vi "ScreenshotSingleVIs.vi"(6 "Title Prefix In":string, 8 "error in":errorcluster, 9 "Picture Save Location":path, 10 "New VI Path":path) -> (0 "error out":errorcluster)   [LabVIEW 2015, in "VIDiffScreenshots.lvlib"]
uses:
  VIDiffScreenshots.lvlib
  Utilities/Arguments.ctl
  VIScreenshots.ctl
  ScreenshotInfo.ctl
  Screenshot Type.ctl
  Utilities/FilePaths.ctl
  Utilities/VIDiffUtilities.lvlib
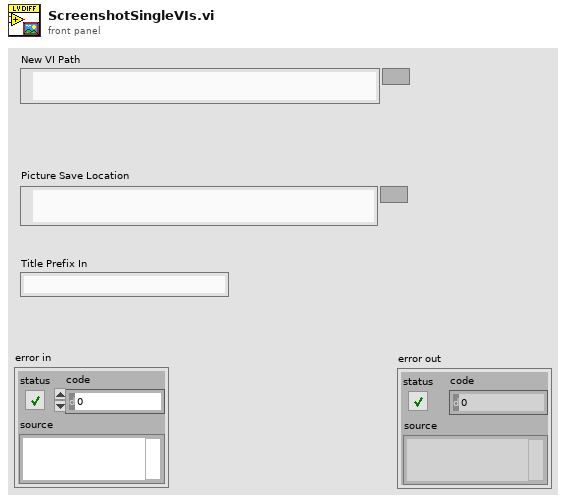
[diagram p1: front panel]
types:
  T1 = typedef "VIDiffScreenshots.lvlib/Screenshot Type.ctl" = enum16{"Unknown", "Front Panel", "Connector Pane", "Block Diagram", "VI Hierarchy"}
  T2 = typedef "VIDiffScreenshots.lvlib/VIScreenshots.ctl" = cluster{"Front Panel Screenshots":T3[], "Block Diagram Screenshots":T3[], "Connector Pane Screenshots":T3[], "VI Hierarchy Screenshots":T3[], "Unknown Screenshots":T3[], "vi reference":refnum<vi>, "File Paths":cluster{"File Path":path}, "Name":string}
  T3 = typedef "VIDiffScreenshots.lvlib/ScreenshotInfo.ctl" = cluster{"Screenshot Path":path, "Screenshot Type":T1, "VI Paths":T4}
  T4 = typedef "VIDiffUtilities.lvlib/FilePaths.ctl" = cluster{"File Path":path}
  T5 = typedef "VIDiffUtilities.lvlib/Arguments.ctl" = cluster{"VI 1 Path":path, "VI 2 Path":path, "Picture Save Location":path, "Screenshot Title":string}
  T6 = typedef "VIDiffUtilities.lvlib/Output Folders.ctl" = cluster{"combined":path, "vi1shots":path, "vi2shots":path, "Picture Save Location":path}
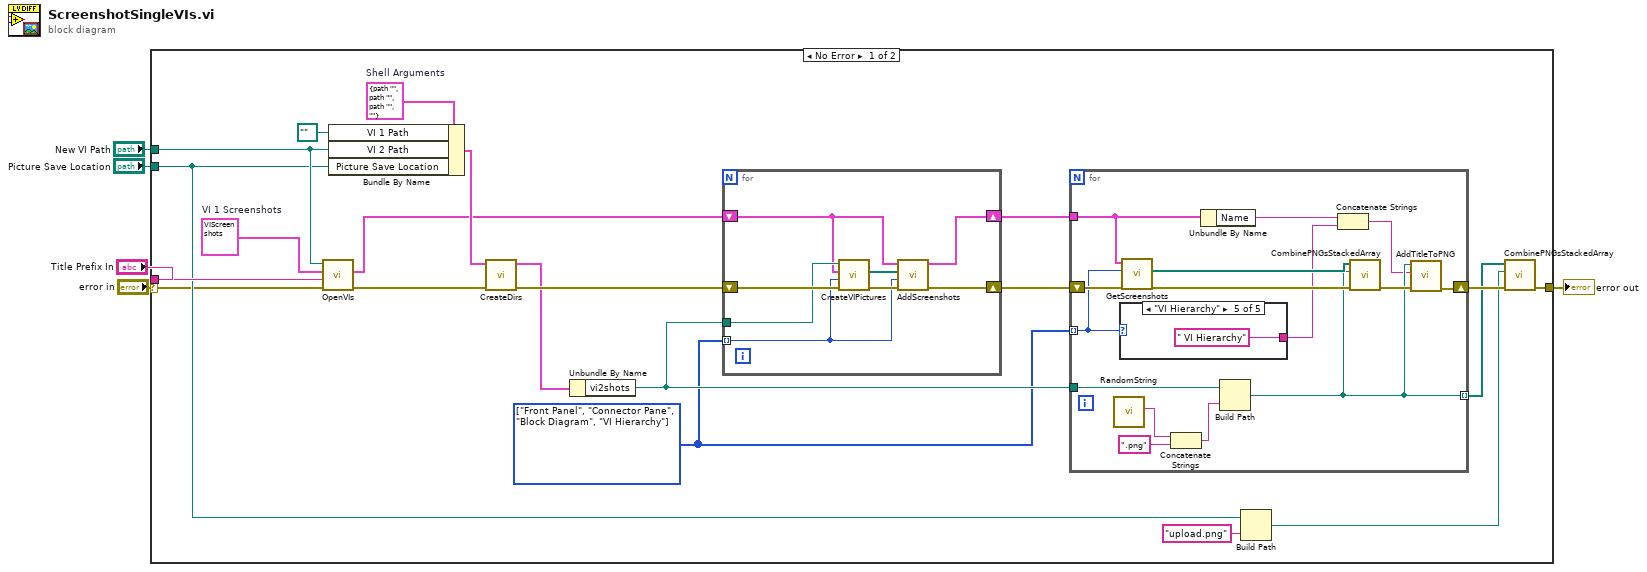
[diagram p0: block diagram]
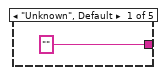
[diagram p2: hidden frame]
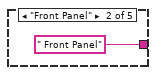
[diagram p3: hidden frame]
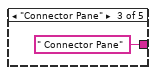
[diagram p4: hidden frame]
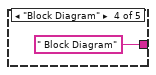
[diagram p5: hidden frame]
diagram:
  n1 = case shown="No Error" "error in" {
    selector: "error in" -> [w6 w55]
    tunnel: "Title Prefix In" -> [w20 _]
    tunnel: "New VI Path" -> [w13 _]
    tunnel: [w11 w55] -> w3
    tunnel: "Picture Save Location" -> [w8 _]
    frame No Error {
      w15 = T1[] [enum."Front Panel", enum."Connector Pane", enum."Block Diagram", enum."VI Hierarchy"] items=["Unknown", "Front Panel", "Connector Pane", "Block Diagram", "VI Hierarchy"]
      w24 = T2 {"Front Panel Screenshots"=[], "Block Diagram Screenshots"=[], "Connector Pane Screenshots"=[], "VI Hierarchy Screenshots"=[], "Unknown Screenshots"=[], "vi reference"=refnum, "File Paths"={"File Path"=path ""}, "Name"=""}  # VI 1 Screenshots
      w26 = T5 {"VI 1 Path"=path "", "VI 2 Path"=path "", "Picture Save Location"=path "", "Screenshot Title"=""}  # Shell Arguments
      n2 = call "OpenVIs.vi"("error in (no error)"=w6, "Title Prefix In"=w20, "VI Screenshots"=w24, "VI Path"=w13) -> ("error out"=w19:errorcluster, "VI Screenshots out"=w23:T2)  [unwired: 6 in]
      n3 = Bundle By Name(cluster=w26, "VI 1 Path"=path "" ("VI Path 2"), "VI 2 Path"=w13, "Picture Save Location"=w8) -> (w25:T5)
      n4 = call "CreateDirs.vi"("error in (no error)"=w19, "Shell Arguments"=w25) -> ("error out"=w22:errorcluster, "Output Folders"=w21:T6)  [unwired: 8 in]
      n5 = Unbundle By Name(w21) -> ("vi2shots"=w17:path)
      n6 = for {
        tunnel: w15 -> [w48] mode=indexing
        shift-right: [w47] -> w16
        shift-left: w22 -> [w54]
        tunnel: w17 -> [w53]
        shift-right: [w51] -> w18
        shift-left: w23 -> [w50]
        n7 = call "CreateVIPictures.vi"("error in (no error)"=w54, "Capture Target"=w48, "VI 1 Screenshots"=w50, "Picture Save Location"=w53) -> ("error out"=w49:errorcluster, "Screenshot Files"=w52:path[])  [unwired: 6 in]
        n8 = call "AddScreenshots.vi"("error in (no error)"=w49, "Screenshot Type"=w48, "Screenshot Paths"=w52, "VI Screenshots In"=w50) -> ("error out"=w47:errorcluster, "VI Screenshots Out"=w51:T2)  [unwired: 6 in]
      }
      n9 = for {
        tunnel: w18 -> [w33]
        tunnel: w17 -> [w38]
        tunnel: w15 -> [w29] mode=indexing
        shift-right: [w32] -> w12
        shift-left: w16 -> [w37]
        tunnel: [w31] -> w10 mode=indexing
        n10 = call "RandomString.vi"() -> ("Random String"=w41:string)  [unwired: 11 in]
        n11 = case shown="\"VI Hierarchy\"" w29 {
          tunnel: ["" " Front Panel" " Connector Pane" " Block Diagram" " VI Hierarchy"] -> w30
          frame "Unknown", Default {
          }
          frame "Front Panel" {
          }
          frame "Connector Pane" {
          }
          frame "Block Diagram" {
          }
          frame "VI Hierarchy" {
          }
        }
        n12 = call "GetScreenshots.vi"("error in (no error)"=w37, "Screenshot Type"=w29, "VI Screenshots In"=w33) -> ("error out"=w35:errorcluster, "Screenshot Paths"=w36:path[])  [unwired: 7 in]
        n13 = Concatenate Strings(w41, ".png" ("string")) -> (w39:string)
        n14 = Unbundle By Name(w33) -> ("Name"=w28:string)
        n15 = Build Path(base path=w38, name or relative path=w39) -> (appended path=w31:path)
        n16 = Concatenate Strings(w28, w30) -> (w27:string)
        n17 = call "CombinePNGsStackedArray.vi"("error in (no error)"=w35, "Output File"=w31, "Input Files"=w36) -> ("error out"=w34:errorcluster)  [unwired: 8 in]
        n18 = call "AddTitleToPNG.vi"("error in (no error)"=w34, "Title String"=w27, "PNG File"=w31) -> ("error out"=w32:errorcluster)  [unwired: 8 in]
      }
      n19 = Build Path(base path=w8, name or relative path="upload.png") -> (appended path=w7:path)
      n20 = call "CombinePNGsStackedArray.vi"("error in (no error)"=w12, "Output File"=w7, "Input Files"=w10) -> ("error out"=w11:errorcluster)  [unwired: 8 in]
    }
    frame Error {
    }
  }
  "error out" <- w3
